vi "Write Power FIFO.vi"(6 "FIFO Timestamps":T1, 8 "error in (no error)":errorcluster, 9 "Timeout (ms)":i32=100, 10 "Data In":T2[](array[typedef])=[{"measurement"=[], "dT"=0.0, "Timestamp"=0, "Read Lock"=FALSE}, {"measurement"=[], "dT"=0.0, "Timestamp"=0, "Read Lock"=FALSE}], 11 "CIFTag in":refnum<class "CIF_NIChn_Fifo_Power.lvclass">) -> (0 "error out":errorcluster, 1 "timed out?":bool, 2 "Data Out":T2[](array[typedef]), 3 "CIFTag out":refnum<class "CIF_NIChn_Fifo_Power.lvclass">)   [LabVIEW 2021, in "CIF_NIChn_Fifo_Power.lvclass"]
uses:
  CIF_NIChn_Fifo_Power.lvclass
  D:/dev/Packages/Channel_Manager/src/CIFChannels/CIFChannels.lvclass
  D:/dev/Packages/Channel_Manager/src/CIF_NIChn/NIChn/CIF_NIChn.lvclass
  ChannelCommon/typedef/Datatype Waveform.ctl
  ChannelCommon/typedef/TimeStamps.ctl
  CIF_NIChn_Fifo_Power.lvclass/CIF_NIChn_Fifo_Power.ctl
  CIFChannels/CIFChannels.lvclass/CIFChannels.ctl
  NIChn/CIF_NIChn.lvclass/CIF_NIChn.ctl
  CIFChannels/Accessors/Read FIFO Payload Length.vi
  <vilib>/CIF Foundation/CIF Utilities/Errors/Append Error Location.vi
  <vilib>/CIF Foundation/CIF Channels/CIFChannels/SubVIs/Get dll Path.vi
  <vilib>/CIF Foundation/CIF Channels/CIFChannels/SubVIs/Get Requested Size.vi
  ChannelCommon/CIFFIFO/Flatten/Waveform Flatten.vi
  <vilib>/CIF Foundation/CIF Utilities/DataTypes/Flatten I64.vi
  ChannelCommon/CIFFIFO/Flatten/Waveform Flatten.vi/be24e584-1bb9-4ddb-b1ad-5fa4498d0a1e.vi
  <vilib>/CIF Foundation/CIF Utilities/DataTypes/Flatten U64.vi
  CIFChannels/Utilities/Create Flattened FIFO Header.vi
  ChannelCommon/CIFFIFO/Flatten/Waveform Flatten.vi/be24e584-1bb9-4ddb-b1ad-5fa4498d0a1e.vi/c28b0ead-42ad-4072-80a2-aca7f2bd7ce3.vi
  ChannelCommon/Utilities/Flatten Header.vi
  CIFChannels/Utilities/Update FIFO Header.vi
  <vilib>/CIF Foundation/CIF Utilities/Time/System Time/Get System Time.vi
  <vilib>/CIF Foundation/CIF Utilities/Time/System Time/LabVIEW Time to TAI Time.vi
  NIChn/CIF_NIChn.lvclass
  <vilib>/CIF Foundation/CIF Channels/CIFChannels/CIFChannelCore.lvlib
  ChannelCommon/ChannelCommon.lvlib
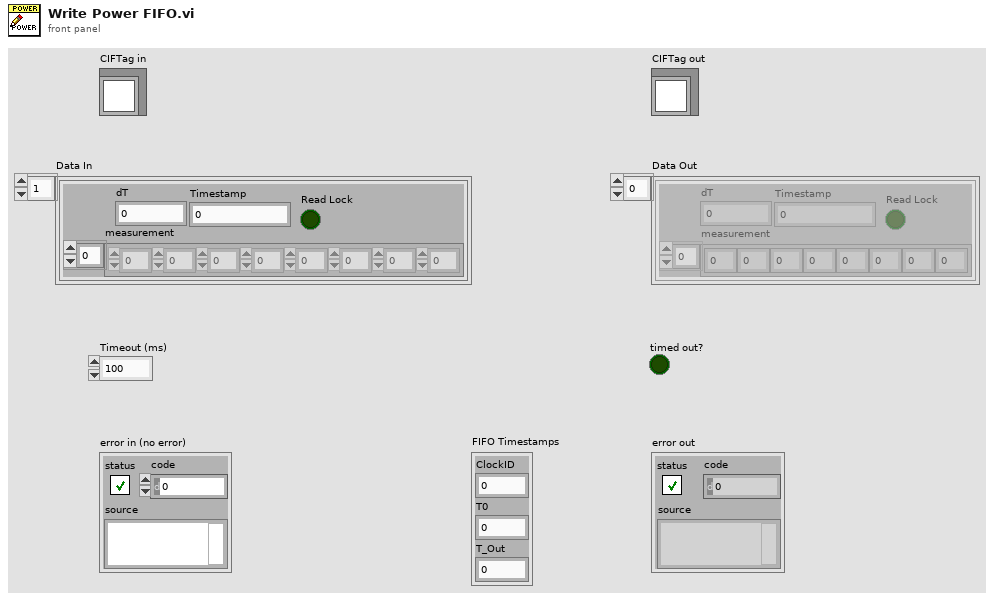
[diagram p1: front panel]
types:
  T1 = typedef "ChannelCommon.lvlib/TimeStamps.ctl" = cluster{"ClockID":u8, "T0":i64, "T_Out":i64}
  T2 = typedef "ChannelCommon.lvlib/Datatype Waveform.ctl" = cluster{"measurement":dbl[], "dT":dbl, "Timestamp":i64, "Read Lock":bool}
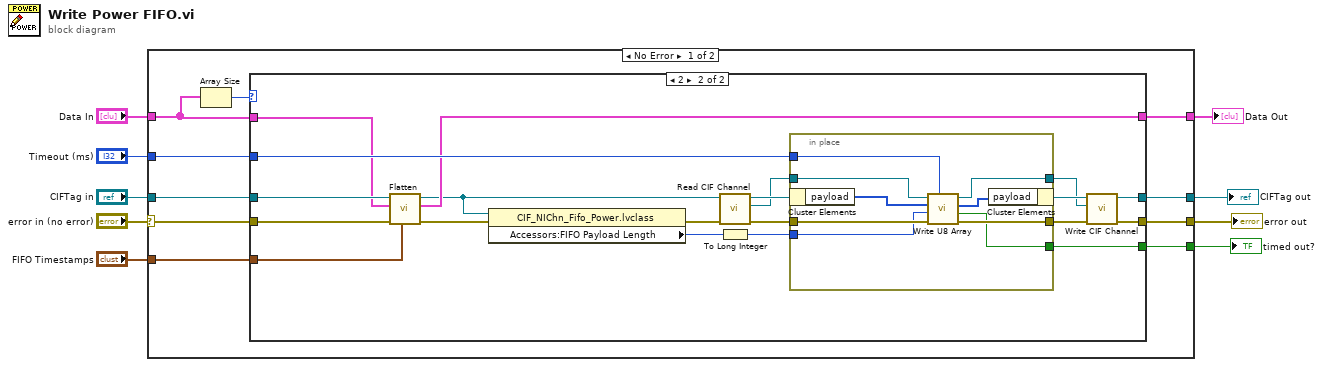
[diagram p0: block diagram]
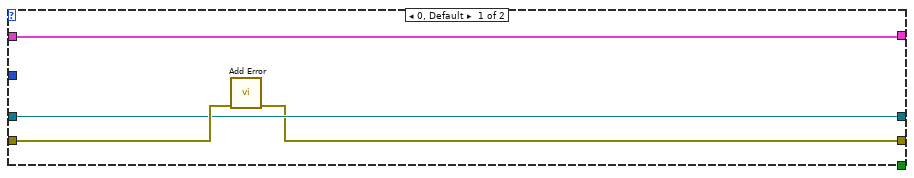
[diagram p2: hidden frame]
diagram:
  n1 = case shown="No Error" "error in (no error)" {
    selector: "error in (no error)" -> [w14 w55]
    tunnel: [w16 w55] -> w8
    tunnel: [w18 w54] -> w6
    tunnel: "CIFTag in" -> [w15 w54]
    tunnel: [w19 _] -> w5
    tunnel: "Timeout (ms)" -> [w17 _]
    tunnel: [w13 w53] -> w3
    tunnel: "Data In" -> [w12 w53]
    tunnel: "FIFO Timestamps" -> [w10 _]
    frame No Error {
      n2 = Array Size(array=w12) -> (size(s)=w11:i32)
      n3 = case shown="2" w11 {
        tunnel: [_ w43] -> w19
        tunnel: [w22 w39] -> w18
        tunnel: w17 -> [_ w35]
        tunnel: [w21 w34] -> w16
        tunnel: w15 -> [w22 w32]
        tunnel: w14 -> [w23 w30]
        tunnel: [w20 w28] -> w13
        tunnel: w12 -> [w20 w27]
        tunnel: w10 -> [_ w26]
        frame 0, Default {
          n4 = call "Add Error.vi"("error in (no error)"=w23) -> ("error out"=w21:errorcluster)  [unwired: 10 in]
        }
        frame 2 {
          n5 = call "Flatten.vi"("FIFO Timestamps"=w26, "error in (no error)"=w30, "Data"=w27, "CIFTag in"=w32) -> ("error out"=w31:errorcluster, "Data out"=w28:T2[], "CIFTag out"=w25:refnum<class "CIF_NIChn_Fifo_Power.lvclass">)  [unwired: 5 in]
          n6 = property class="CIF_NIChn_Fifo_Power.lvclass"(reference=w25, error in=w31) -> (error out=w33:errorcluster, "Accessors:FIFO Payload Length"=w29:u64)  [unwired: 1 out]
          n7 = call "Read CIF Channel.vi"("error in (no error)"=w33, "CIFTag in"=w25) -> ("error out"=w41:errorcluster, "CIF Channel"=w37:refnum<k21>, "CIFTag out"=w42:refnum<class "CIF_NIChn_Fifo_Power.lvclass">)  [unwired: 7 in]
          n8 = To Long Integer(number=w29) -> (32bit integer=w24:i32)
          n9 = in-place {
            in-place-border: w41 -> [w52]
            in-place-border: [w51] -> w38
            in-place-border: [w50] -> w43
            in-place-border: w37 -> [w49]
            in-place-border: [w48] -> w36
            in-place-border: w35 -> [w47]
            in-place-border: w24 -> [w45]
            n10 = in-place-cluster #1(w42) -> ("payload"=w46:u8[])
            n11 = call <vilib>:"Write U8 Array.vi"("Timeout (ms)"=w47, "error in"=w52, "Number of Elements"=w45, "U8 Array in"=w46, "CIF Channel in"=w49) -> ("error out"=w51:errorcluster, "Timed out?"=w50:bool, "U8 Array out"=w44:u8[], "CIF Channel out"=w48:refnum<k21>)  [unwired: 3 in]
            n12 = in-place-cluster #1("payload"=w44) -> (w40:refnum<class "CIF_NIChn_Fifo_Power.lvclass">)
          }
          n13 = call "Write CIF Channel.vi"("error in (no error)"=w38, "CIF Channel"=w36, "CIFTag in"=w40) -> ("error out"=w34:errorcluster, "CIFTag out"=w39:refnum<class "CIF_NIChn_Fifo_Power.lvclass">)  [unwired: 7 in]
        }
      }
    }
    frame Error {
    }
  }
  "error out" <- w8
  "CIFTag out" <- w6
  "timed out?" <- w5
  "Data Out" <- w3
